vi "Update State Data.vi"(8 "error in (no error)":errorcluster, 9 "Data":variant, 10 "Argument":string, 11 "Keyboard Action in":refnum<class "Keyboard Action.lvclass">) -> (0 "error out":errorcluster, 3 "Keyboard Action out":refnum<class "Keyboard Action.lvclass">)   [LabVIEW 2020, in "MacroAssert.lvlib" / "Keyboard Action.lvclass"]
uses:
  Keyboard Action.lvclass
  Keyboard Action Type.ctl
  Action Step/Action Step.lvclass
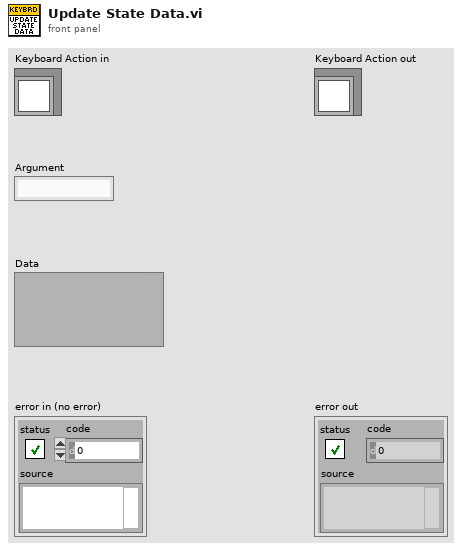
[diagram p1: front panel]
types:
  T1 = typedef "MacroAssert.lvlib/Keyboard Action.lvclass/Keyboard Action Type.ctl" = enum16{"Key Press", "Key Down", "Key Up"}
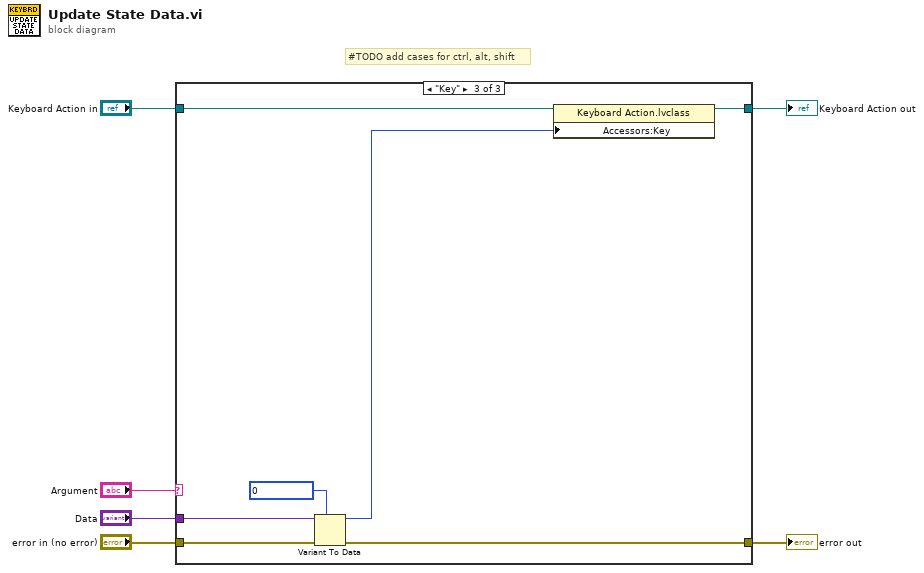
[diagram p0: block diagram]
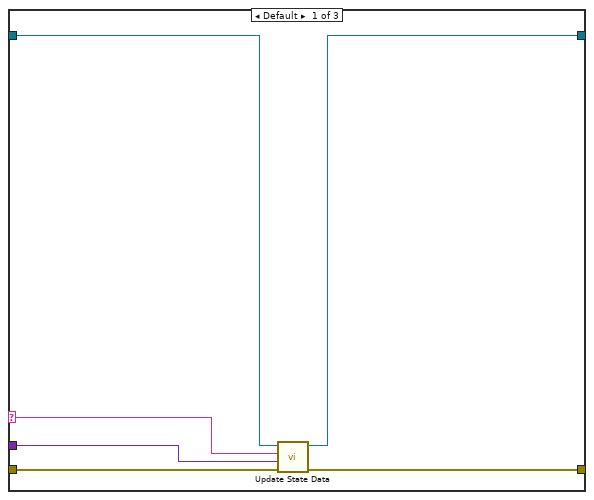
[diagram p2: hidden frame]
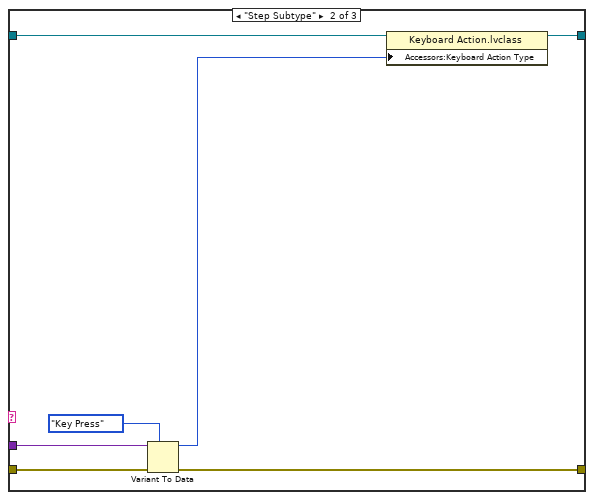
[diagram p3: hidden frame]
diagram:
  # "#TODO add cases for ctrl, alt, shift"
  n1 = case shown="\"Key\"" "Argument" {
    selector: "Argument" -> [w9 _ _]
    tunnel: "Keyboard Action in" -> [w8 w19 w26]
    tunnel: "error in (no error)" -> [w12 w17 w24]
    tunnel: [w7 w18 w25] -> w3
    tunnel: [w11 w16 w23] -> w5
    tunnel: "Data" -> [w10 w14 w22]
    frame Default {
      n2 = call-parent "Update State Data.vi"("error in (no error)"=w12, "Data"=w10, "Argument"=w9, "Step in"=w8) -> ("error out"=w11:errorcluster, "Step out"=w7:refnum<class "Keyboard Action.lvclass">)  [unwired: 6 in]
    }
    frame "Step Subtype" {
      n3 = Variant To Data(error in=w17, type=Keyboard_Action_Type."Key Press" ("Keyboard Action Type"), Variant=w14) -> (data=w13:T1, error out=w16:errorcluster)
      n4 = property class="Keyboard Action.lvclass"(reference=w19, "Accessors:Keyboard Action Type"=w13) -> (reference out=w18:refnum<class "Keyboard Action.lvclass">)  [unwired: 1 in, 1 out]
    }
    frame "Key" {
      n5 = Variant To Data(error in=w24, type=u8 0 ("Key"), Variant=w22) -> (data=w20:u8, error out=w23:errorcluster)
      n6 = property class="Keyboard Action.lvclass"(reference=w26, "Accessors:Key"=w20) -> (reference out=w25:refnum<class "Keyboard Action.lvclass">)  [unwired: 1 in, 1 out]
    }
  }
  "error out" <- w5
  "Keyboard Action out" <- w3
